vi "CreateEvent.vi"(0 "Shared Variable":refnum<k21>[](array[refnum]), 1 "TypeDescriptor":string[](array[string]), 2 "Command(t)/\nSubscriber(f)":bool[](array[boolean]), 3 "InitValue":string[](array[string]), 5 "error in (no error)":errorcluster, 8 "HGF_Event (Monitor Event)":refnum<class "HGF_Event.lvclass">) -> (16 "HGF Event":refnum<class "HGF_Event.lvclass">, 19 "error out":errorcluster)   [LabVIEW 2012, in "HGF_DSC.lvlib" / "HGF_DSCEvent.lvclass"]
uses:
  HGF_DSCEvent.lvclass
  HGF_BaseClasses/HGF_Event/HGF_Event.lvclass
  HGF_DSCFactory/HGF_DSCFactory.lvclass
  HGF_SV/HGF_SVDataConverter/HGF_SVDataConverter.lvclass
  HGF_BaseClasses/HGF_PVSubscriber/HGF_PVSubscriber.lvclass
  HGF_BaseClasses/HGF_NetworkVisitor/HGF_NetworkVisitor.lvclass
  HGF_DSCCommand/HGF_DSCCommand.lvclass
  HGF_DSCSubscriber/HGF_DSCSubscriber.lvclass
  HGF_BaseClasses/HGF_Factory/HGF_Factory.lvclass
  HGF_BaseClasses/HGF_NetworkEvent/HGF_NetworkEvent.lvclass/HGF_NetworkEvent.lvclass
  HGF_BaseClasses/HGF_PVBase/HGF_PVBase.lvclass
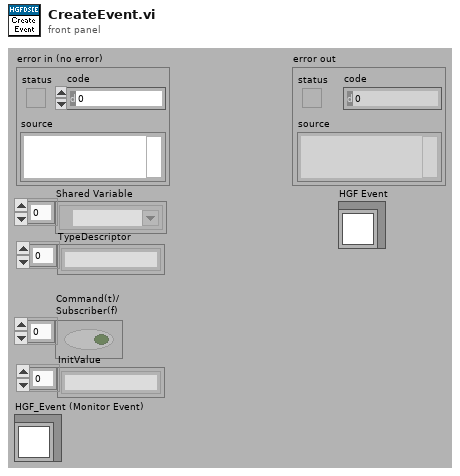
[diagram p1: front panel]
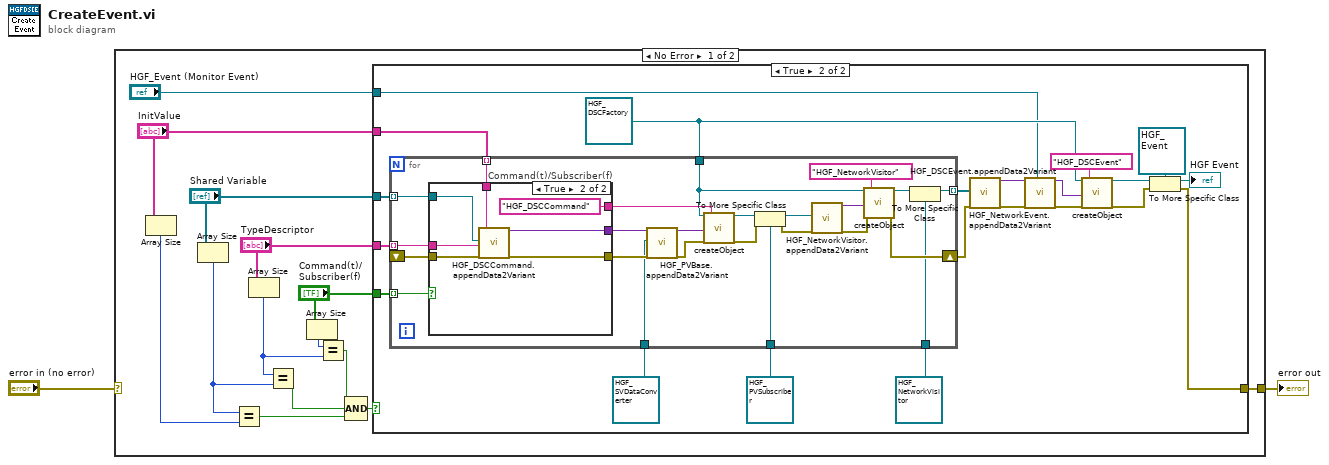
[diagram p0: block diagram]
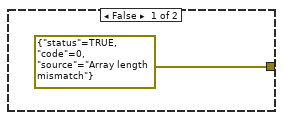
[diagram p2: hidden frame]
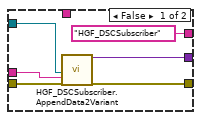
[diagram p3: hidden frame]
diagram:
  n1 = case shown="No Error" "error in (no error)" {
    selector: "error in (no error)" -> [_ w76]
    tunnel: [w4 w76] -> w1
    frame No Error {
      n2 = Array Size(array="InitValue") -> (size(s)=w11:i32)
      n3 = Array Size(array="Shared Variable") -> (size(s)=w9:i32)
      n4 = Equal?(x=w9, y=w11) -> (x = y?=w6:bool)
      n5 = Array Size(array="TypeDescriptor") -> (size(s)=w10:i32)
      n6 = Equal?(x=w10, y=w9) -> (x = y?=w7:bool)
      n7 = Array Size(array="Command(t)/\nSubscriber(f)") -> (size(s)=w12:i32)
      n8 = Equal?(x=w12, y=w10) -> (x = y?=w8:bool)
      n9 = Compound Arithmetic op=AND(w8, w7, w6) -> (w5:bool)
      n10 = case shown="True" w5 {
        tunnel: "InitValue" -> [_ w38]
        tunnel: "Shared Variable" -> [_ w37]
        tunnel: "TypeDescriptor" -> [_ w36]
        tunnel: "Command(t)/\nSubscriber(f)" -> [_ w35]
        tunnel: "HGF_Event (Monitor Event)" -> [_ w18]
        tunnel: [errorcluster {"status"=TRUE, "code"=0, "source"="Array length mismatch"} ("error out") w20] -> w4
        frame False {
        }
        frame True {
          w25 = refnum<class "HGF_DSCFactory.lvclass"> refnum ("DSC.lvlib:HGF_DSCFactory.lvclass")
          n11 = for {
            tunnel: w38 -> [w62] mode=indexing
            tunnel: w37 -> [w61] mode=indexing
            tunnel: w36 -> [w60] mode=indexing
            tunnel: w35 -> [w59] mode=indexing
            tunnel: w25 -> [w45]
            shift-right: [w43] -> w30
            shift-left: _ -> [w55]
            tunnel: refnum<class "HGF_SVDataConverter.lvclass"> refnum ("HGF_SV.lvlib:HGF_SVDataConverter.lvclass") -> [w51]
            tunnel: refnum<class "HGF_PVSubscriber.lvclass"> refnum ("HGF_BaseClasses.lvlib:HGF_PVSubscriber.lvclass") -> [w49]
            tunnel: [w39] -> w31 mode=indexing
            tunnel: refnum<class "HGF_NetworkVisitor.lvclass"> refnum ("HGF_BaseClasses.lvlib:HGF_NetworkVisitor.lvclass") -> [w40]
            n12 = case "Command(t)/Subscriber(f)" shown="True" w59 {
              tunnel: w62 -> [_ w75]
              tunnel: w61 -> [w66 w74]
              tunnel: w60 -> [w65 w73]
              tunnel: ["HGF_DSCSubscriber" "HGF_DSCCommand"] -> w58
              tunnel: [w67 w71] -> w53
              tunnel: w55 -> [w64 w70]
              tunnel: [w63 w69] -> w52
              frame False {
                n13 = call "HGF_DSCSubscriber.AppendData2Variant.vi"("Shared Variable"=w66, "TypeDescriptor"=w65, "error in"=w64) -> ("variant out"=w67:variant, "error out"=w63:errorcluster)  [unwired: 1 in, 14 out]
              }
              frame True {
                n14 = call "HGF_DSCCommand.appendData2Variant.vi"("SV"=w74, "typeDescriptor"=w73, "error in (no error)"=w70, "initValue"=w75) -> ("dup initData"=w71:variant, "error out"=w69:errorcluster)  [unwired: 1 in, 13 out]
              }
            }
            n15 = call "HGF_PVBase.appendData2Variant.vi"("initData"=w53, "HGF_PVDataConverter"=w51, "error in (no error)"=w52) -> ("dup initData"=w54:variant, "error out"=w50:errorcluster)  [unwired: 15 out]
            n16 = call "createObject.vi"("HGF_Factory"=w45, "initializationData"=w54, "error in (no error)"=w50, "className"=w58) -> ("HGF_Object"=w56:refnum<class "HGF_Factory.lvclass">, "error out"=w57:errorcluster)  [unwired: 1 in, 13 out]
            n17 = To More Specific Class(target class=w49, reference=w56, error in=w57) -> (specific class reference=w48:refnum<class "HGF_PVSubscriber.lvclass">, error out=w47:errorcluster)
            n18 = call "HGF_NetworkVisitor.appendData2Variant.vi"("HGF_PVSubscriber"=w48, "error in (no error)"=w47) -> ("dup initData"=w46:variant, "error out"=w44:errorcluster)  [unwired: 1 in, 15 out]
            n19 = call "createObject.vi"("HGF_Factory"=w45, "initializationData"=w46, "error in (no error)"=w44, "className"="HGF_NetworkVisitor") -> ("HGF_Object"=w41:refnum<class "HGF_Factory.lvclass">, "error out"=w43:errorcluster)  [unwired: 1 in, 13 out]
            n20 = To More Specific Class(target class=w40, reference=w41) -> (specific class reference=w39:refnum<class "HGF_NetworkVisitor.lvclass">)  [unwired: 1 in, 1 out]
          }
          n21 = call "HGF_NetworkEvent.appendData2Variant.vi"("callbackVisitors"=w31, "error in (no error)"=w30) -> ("dup initData"=w28:variant, "error out"=w29:errorcluster)  [unwired: 1 in, 15 out]
          n22 = call "HGF_DSCEvent.appendData2Variant.vi"("initData"=w28, "error in (no error)"=w29, "HGF_Event (Monitor Event)"=w18) -> ("dup initData"=w27:variant, "error out"=w26:errorcluster)  [unwired: 1 in, 14 out]
          n23 = call "createObject.vi"("HGF_Factory"=w25, "initializationData"=w27, "error in (no error)"=w26, "className"="HGF_DSCEvent") -> ("HGF_Object"=w23:refnum<class "HGF_Factory.lvclass">, "error out"=w22:errorcluster)  [unwired: 1 in, 13 out]
          n24 = To More Specific Class(target class=refnum<class "HGF_Event.lvclass"> refnum ("HGF_BaseClasses.lvlib:HGF_Event.lvclass"), reference=w23, error in=w22) -> (specific class reference=→"HGF Event":refnum<class "HGF_Event.lvclass">, error out=w20:errorcluster)
        }
      }
    }
    frame Error {
    }
  }
  "error out" <- w1
